vi "Control Intake.vi"(11 "Avoid Race Condition":bool) -> ()   [LabVIEW 2020]
uses:
  Framework/Robot Global Data.vi
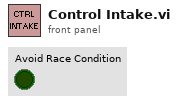
[diagram p1: front panel]
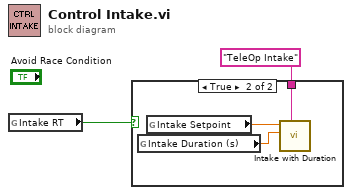
[diagram p0: block diagram]
diagram:
  n1 = global read "Robot Global Data.vi" "Intake RT"() -> (w2:bool)
  n2 = case shown="True" w2 {
    tunnel: "TeleOp Intake" ("Description") -> [_ w3]
    frame False {
    }
    frame True {
      n3 = global read "Robot Global Data.vi" "Intake Duration (s)"() -> (w4:dbl)
      n4 = global read "Robot Global Data.vi" "Intake Setpoint"() -> (w5:dbl)
      n5 = call "Intake with Duration.vi"("Description"=w3, "Duration (s)"=w4, "Setpoint"=w5) -> ()  [unwired: 8 in, 1 out]
    }
  }
